vi "Helper - InterpretKeyPress.vi"(4 "Sail Key Control Config":T4={"Sail Position Max"=1.0, "Sail Position Increment"=0.01}, 6 "Rudder Key Control Config":T2={"Rudder Angle Max"=50.0, "Rudder Angle Increment"=1.0}, 9 "VKey":T1=enum."Up", 10 "Char":i16, 11 "Command In":T6={"Sail Position"=0.0, "Rudder Angle"=6.0}) -> (3 "Command Out":T6={"Sail Position"=0.0, "Rudder Angle"=6.0})   [LabVIEW 2011]
doc: "Update sailboat commands (rudder angle and sail position currently) according to key presses. Configuration options are exposed which allow the upper range of the value to be selected and the increment associated with the appropriate key press.\n\nAssumptions:\n- the minimum value for all commands is 0\n\nAuthor: Jared Kirschner"
uses:
  2-Think/2 Typedefs/setpoints to boat.ctl
  2-Think/2 Typedefs/sail setpt.ctl
  2-Think/2 Typedefs/rudder angle.ctl
  0 Typedefs/sailKeyControlConfig.ctl
  0 Typedefs/rudderKeyControlConfig.ctl
  <vilib>/event_ctls.llb/eventvkey.ctl
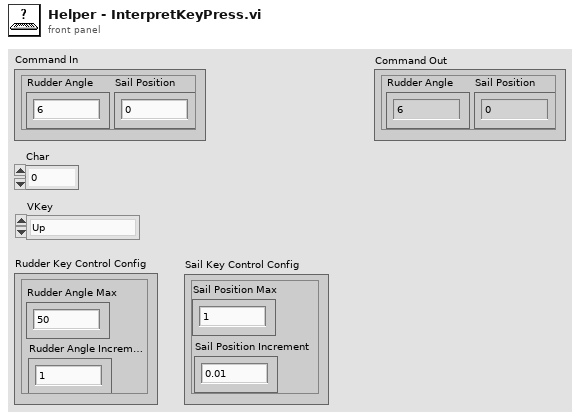
[diagram p1: front panel]
types:
  T1 = typedef "eventvkey.ctl" = enum16{"ASCII", "Enter", "Return", "Shift", "Ctrl", "Alt", "Cmd", "Opt", "Caps", "NumLock", "Clear", "Break", "Up", "Down", "Left", "Right", "Insert", "Delete", "Home", "End", "PageUp", "PageDown", "Escape", "Help", "Pause", "ScrollLock", "F1", "F2", "F3", "F4", "F5", "F6", "F7", "F8", "F9", "F10", "F11", "F12", "F13", "F14", "F15", "F16", "F17", "F18", "F19", "F20", "F21", "F22", "F23", "F24", "Play", "VolumeUp", "VolumeDown", "Mute", "Two Byte Char"}
  T2 = typedef "rudderKeyControlConfig.ctl" = cluster{"Rudder Angle Max":T3, "Rudder Angle Increment":T3}
  T3 = typedef "rudder angle.ctl" = dbl
  T4 = typedef "sailKeyControlConfig.ctl" = cluster{"Sail Position Max":T5, "Sail Position Increment":T5}
  T5 = typedef "sail setpt.ctl" = dbl
  T6 = typedef "setpoints to boat.ctl" = cluster{"Sail Position":T5, "Rudder Angle":T3}
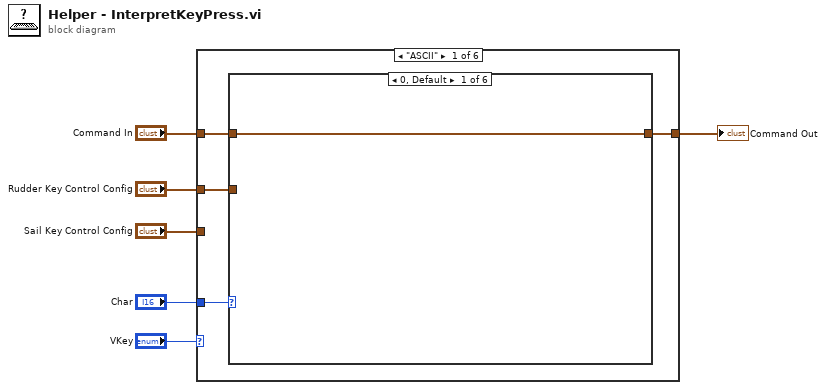
[diagram p0: block diagram]
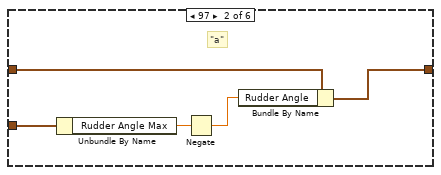
[diagram p2: hidden frame]
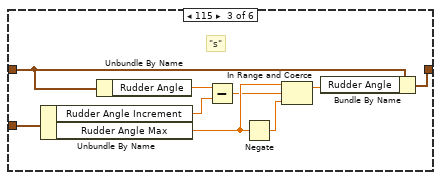
[diagram p3: hidden frame]
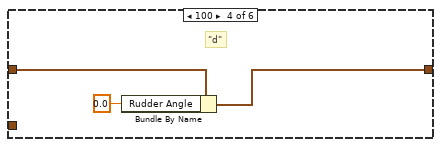
[diagram p4: hidden frame]
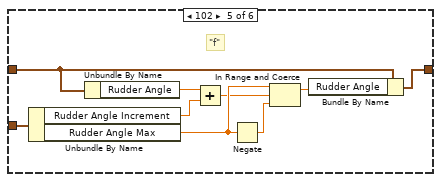
[diagram p5: hidden frame]
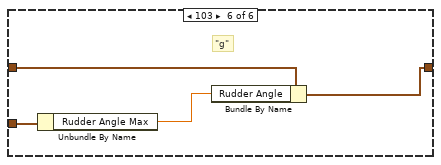
[diagram p6: hidden frame]
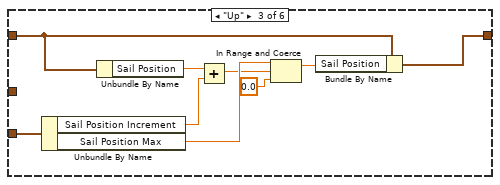
[diagram p8: hidden frame]
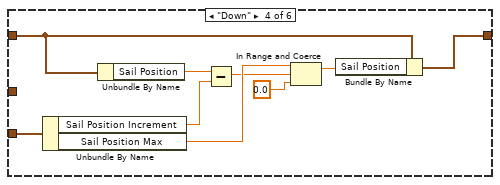
[diagram p9: hidden frame]
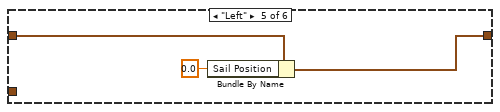
[diagram p10: hidden frame]
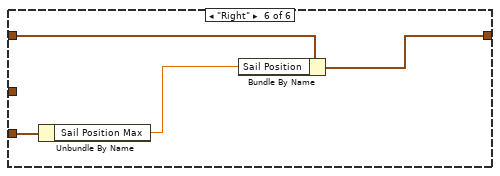
[diagram p11: hidden frame]
diagram:
  n1 = case shown="\"ASCII\"" "VKey" {
    tunnel: "Command In" -> [w9 w42 w44 w54 w62 w65]
    tunnel: "Rudder Key Control Config" -> [w7 _ _ _ _ _]
    tunnel: "Sail Key Control Config" -> [_ _ w45 w53 _ w66]
    tunnel: "Char" -> [w10 _ _ _ _ _]
    tunnel: [w8 w42 w43 w52 w61 w64] -> w1
    frame "ASCII" {
      n2 = case shown="0, Default" w10 {
        tunnel: w9 -> [w11 w14 w18 w27 w30 w39]
        tunnel: [w11 w13 w17 w26 w29 w38] -> w8
        tunnel: w7 -> [_ w12 w19 _ w31 w40]
        frame 0, Default {
        }
        frame 97 {
          # "\"a\""
          n3 = Unbundle By Name(w12) -> ("Rudder Angle Max"=w15:T3)
          n4 = Negate(x=w15) -> (-x=w16:T3)
          n5 = Bundle By Name(cluster=w14, "Rudder Angle"=w16) -> (w13:T6)
        }
        frame 115 {
          # "\"s\""
          n6 = Unbundle By Name(w19) -> ("Rudder Angle Increment"=w22:T3, "Rudder Angle Max"=w24:T3)
          n7 = Unbundle By Name(w18) -> ("Rudder Angle"=w20:T3)
          n8 = Subtract(x=w20, y=w22) -> (x-y=w21:T3)
          n9 = Negate(x=w24) -> (-x=w23:T3)
          n10 = In Range and Coerce(upper limit=w24, x=w21, lower limit=w23) -> (coerced(x)=w25:T3)  [unwired: 1 out]
          n11 = Bundle By Name(cluster=w18, "Rudder Angle"=w25) -> (w17:T6)
        }
        frame 100 {
          # "\"d\""
          n12 = Bundle By Name(cluster=w27, "Rudder Angle"=T3 0.0) -> (w26:T6)
        }
        frame 102 {
          # "\"f\""
          n13 = Unbundle By Name(w31) -> ("Rudder Angle Increment"=w34:T3, "Rudder Angle Max"=w36:T3)
          n14 = Unbundle By Name(w30) -> ("Rudder Angle"=w32:T3)
          n15 = Add(x=w32, y=w34) -> (x+y=w33:T3)
          n16 = Negate(x=w36) -> (-x=w35:T3)
          n17 = In Range and Coerce(upper limit=w36, x=w33, lower limit=w35) -> (coerced(x)=w37:T3)  [unwired: 1 out]
          n18 = Bundle By Name(cluster=w30, "Rudder Angle"=w37) -> (w29:T6)
        }
        frame 103 {
          # "\"g\""
          n19 = Unbundle By Name(w40) -> ("Rudder Angle Max"=w41:T3)
          n20 = Bundle By Name(cluster=w39, "Rudder Angle"=w41) -> (w38:T6)
        }
      }
    }
    frame Default {
    }
    frame "Up" {
      n21 = Unbundle By Name(w45) -> ("Sail Position Increment"=w47:T5, "Sail Position Max"=w49:T5)
      n22 = Unbundle By Name(w44) -> ("Sail Position"=w46:T5)
      n23 = Add(x=w46, y=w47) -> (x+y=w48:T5)
      n24 = In Range and Coerce(upper limit=w49, x=w48, lower limit=T5 0.0 ("Sail Position")) -> (coerced(x)=w51:T5)  [unwired: 1 out]
      n25 = Bundle By Name(cluster=w44, "Sail Position"=w51) -> (w43:T6)
    }
    frame "Down" {
      n26 = Unbundle By Name(w53) -> ("Sail Position Increment"=w56:T5, "Sail Position Max"=w58:T5)
      n27 = Unbundle By Name(w54) -> ("Sail Position"=w55:T5)
      n28 = Subtract(x=w55, y=w56) -> (x-y=w57:T5)
      n29 = In Range and Coerce(upper limit=w58, x=w57, lower limit=T5 0.0 ("Sail Position")) -> (coerced(x)=w60:T5)  [unwired: 1 out]
      n30 = Bundle By Name(cluster=w54, "Sail Position"=w60) -> (w52:T6)
    }
    frame "Left" {
      n31 = Bundle By Name(cluster=w62, "Sail Position"=T5 0.0) -> (w61:T6)
    }
    frame "Right" {
      n32 = Unbundle By Name(w66) -> ("Sail Position Max"=w67:T5)
      n33 = Bundle By Name(cluster=w65, "Sail Position"=w67) -> (w64:T6)
    }
  }
  "Command Out" <- w1
